vi "Close.vi"(8 "error in (no error)":errorcluster, 11 "File Upload Controller in":refnum<class "File Upload Controller.lvclass">) -> (0 "error out":errorcluster, 3 "File Upload Controller out":refnum<class "File Upload Controller.lvclass">)   [LabVIEW 2020, in "NI_SFTP.lvlib" / "File Upload Controller.lvclass"]
uses:
  <vilib>/net/SFTP/API/Support/Upload/File/File Upload Controller.lvclass
  <vilib>/net/SFTP/API/Support/Upload/File/File Upload Controller.lvclass/File Upload Controller.ctl
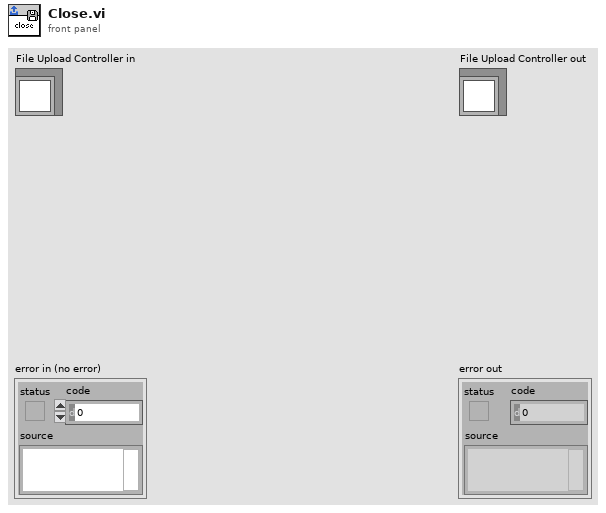
[diagram p1: front panel]
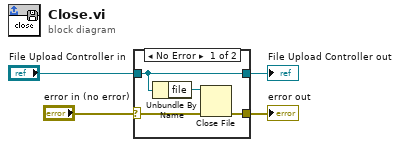
[diagram p0: block diagram]
diagram:
  n1 = case shown="No Error" "error in (no error)" {
    selector: "error in (no error)" -> [w8 w10]
    tunnel: [w6 w10] -> w3
    tunnel: [w7 w9] -> w1
    tunnel: "File Upload Controller in" -> [w7 w9]
    frame No Error {
      n2 = Unbundle By Name(w7) -> ("file"=w5:refnum<file>)
      n3 = Close File(refnum=w5, error in=w8) -> (error out=w6:errorcluster)  [unwired: 1 out]
    }
    frame Error {
    }
  }
  "error out" <- w3
  "File Upload Controller out" <- w1
